vi "Get Main Page Config File Path.vi"(8 "error in":errorcluster, 11 "Main Page Ref in":T1 format="%.0x") -> (0 "error out":errorcluster, 2 "Config File Path":path, 3 "Main Page Ref out":T1 format="%.0x", 4 "Found?":bool)   [LabVIEW 2020, in "afdx_custom_device Scripting.lvlib"]
uses:
  <vilib>/NI VeriStand/Custom Device API/Custom Device Item Ref.ctl
  Constants.vi
  afdx_custom_device Scripting.lvlib
  <vilib>/NI VeriStand/Custom Device API/Get Item Property (Path).vi
  <vilib>/NI VeriStand/Custom Device API/Custom Device API.lvlib
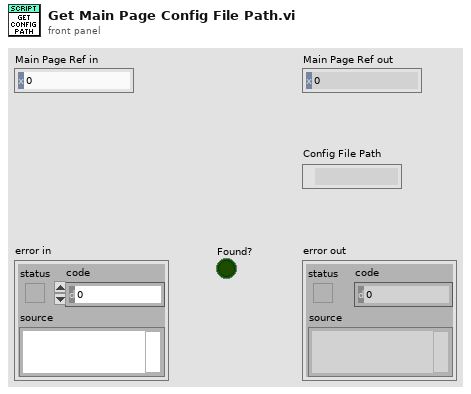
[diagram p1: front panel]
types:
  T1 = typedef "Custom Device API.lvlib/Custom Device Item Ref.ctl" = u64
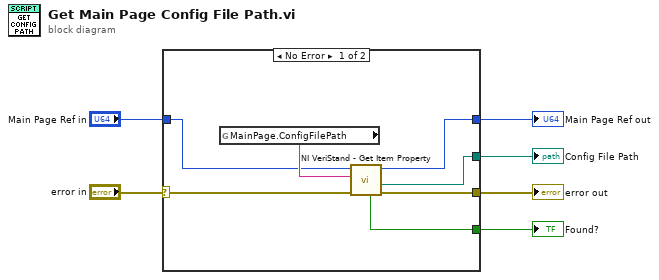
[diagram p0: block diagram]
diagram:
  n1 = case shown="No Error" "error in" {
    selector: "error in" -> [w9 w15]
    tunnel: "Main Page Ref in" -> [w10 w14]
    tunnel: [w13 w15] -> w5
    tunnel: [w12 w14] -> w4
    tunnel: [w8 _] -> w2
    tunnel: [w7 _] -> w1
    frame No Error {
      n2 = global read "Constants.vi" "MainPage.ConfigFilePath"() -> (w11:string)
      n3 = call-poly <vilib>:"NI VeriStand - Get Item Property.vi"("error in (no error)"=w9, "Property Name"=w11, "Item Ref in"=w10) -> ("error out"=w13:errorcluster, "Value"=w8:path, "Item Ref out"=w12:T1, "Found?"=w7:bool)  [unwired: 5 in]
    }
    frame Error {
    }
  }
  "error out" <- w5
  "Config File Path" <- w2
  "Main Page Ref out" <- w4
  "Found?" <- w1
